vi "Write Test File.vi"(10 "Test File":path, 11 "VI Analyzer in":refnum<class "VI Analyzer.lvclass">) -> (3 "VI Analyzer out":refnum<class "VI Analyzer.lvclass">)   [LabVIEW 2014, in "VI Analyzer.lvclass"]
uses:
  VI Analyzer.lvclass
  VI Analyzer.lvclass/VI Analyzer.ctl
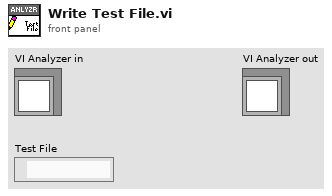
[diagram p1: front panel]
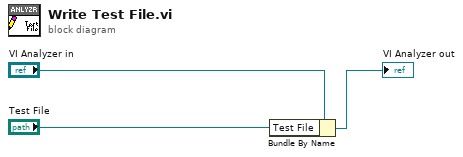
[diagram p0: block diagram]
diagram:
  n1 = Bundle By Name(cluster="VI Analyzer in", "Test File"="Test File") -> (→"VI Analyzer out":refnum<class "VI Analyzer.lvclass">)
